vi "posctrl-drive-spin-sim.vi"(11 "Motor Demand":dbl) -> (3 "Rotation Change Deg":dbl)   [LabVIEW 2019]
uses:
  <vilib>/Rock Robotics/WPI/ThirdParty/JAS_Junk/TrajLib/LinearFilter_LP_BW1_Execute.vi
  <vilib>/Rock Robotics/WPI/ThirdParty/JAS_Junk/TrajLib/VI/TimeInterpDouble_New.vi
  <vilib>/Rock Robotics/WPI/ThirdParty/JAS_Junk/TrajLib/VI/TimeInterpDouble_AddSample.vi
  <vilib>/Rock Robotics/WPI/ThirdParty/JAS_Junk/TrajLib/VI/TimeInterpDouble_GetSample.vi
  <vilib>/Rock Robotics/WPI/ThirdParty/JAS_Junk/TrajLib/VI/TimeInterpDouble_SetMaxTime.vi
  <vilib>/Rock Robotics/WPI/ThirdParty/JAS_Junk/TrajLib/Util_GetTime.vi
  <vilib>/Rock Robotics/WPI/ThirdParty/JAS_Junk/TrajLib/LinearFilter_ResetToValue.vi
  <vilib>/Rock Robotics/WPI/ThirdParty/JAS_Junk/TrajLib/LinearFilter_Calculate.vi
  <vilib>/Rock Robotics/WPI/ThirdParty/JAS_Junk/TrajLib/VI/TimeInterpDouble_CleanUp.vi
  <vilib>/Rock Robotics/WPI/ThirdParty/JAS_Junk/TrajLib/MathUtil_Interpolate.vi
  <vilib>/Rock Robotics/WPI/ThirdParty/JAS_Junk/TrajLib/VI/Util_GetTime_U32.vi
  <vilib>/Rock Robotics/WPI/ThirdParty/JAS_Junk/TrajLib/VI/Util_GetTime_U64.vi
  <vilib>/gmath/interp.llb/Search Ordered Table.vi
  <vilib>/Rock Robotics/WPI/ThirdParty/JAS_Junk/TrajLib/LinearFilter_LowPassBW1.vi
  <vilib>/ptbypt/NI_PtbyPt.lvlib
  <vilib>/Rock Robotics/WPI/ThirdParty/JAS_Junk/TrajLib/Trajectory_Library.lvlib
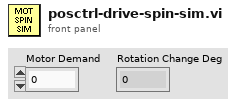
[diagram p1: front panel]
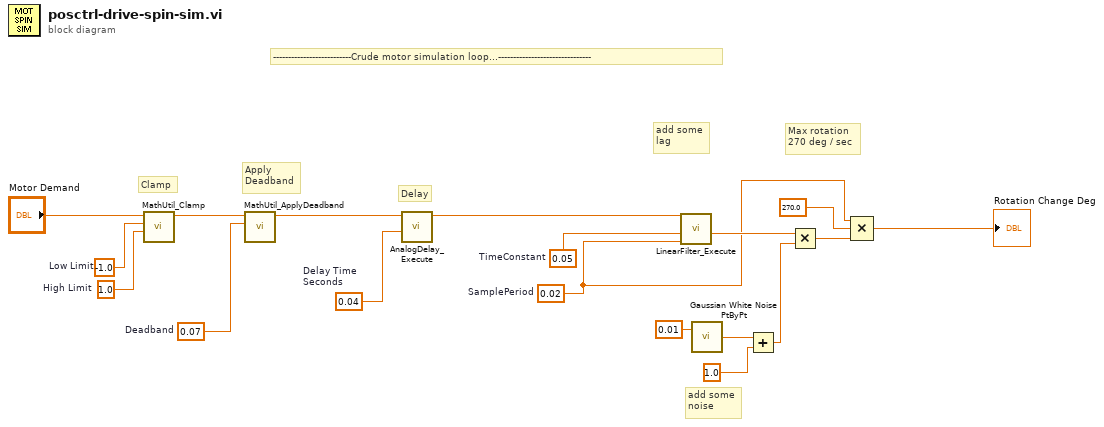
[diagram p0: block diagram]
diagram:
  w5 = 0.07  # Deadband
  w7 = 0.04  # Delay Time Seconds
  w10 = 1.0  # High Limit
  w9 = -1.0  # Low Limit
  w2 = 0.02  # SamplePeriod
  w1 = 0.05  # TimeConstant
  # "Apply\nDeadband"
  # "Delay"
  # "Max rotation \n270 deg / sec"
  # "Clamp"
  # "add some\nnoise"
  # "add some\nlag"
  # "--------------------------Crude motor simulation loop...-------------------------------"
  n1 = call <vilib>:"MathUtil_Clamp.vi"("High Limit"=w10, "Low Limit"=w9, "Value"="Motor Demand") -> ("Result"=w4:dbl)  [unwired: 8 in]
  n2 = call <vilib>:"MathUtil_ApplyDeadband.vi"("Deadband"=w5, "Value"=w4) -> ("Result"=w3:dbl)  [unwired: 9 in]
  n3 = call <vilib>:"AnalogDelay_Execute.vi"("Delay Time"=w7, "Input"=w3) -> ("Output"=w6:dbl)  [unwired: 8 in, 1 out]
  n4 = call-poly <vilib>:"LinearFilter_Execute.vi"("SamplePeriod"=w2, "TimeConstant"=w1, "Input"=w6) -> ("Output"=w14:dbl)  [unwired: 8 in]
  n5 = call <vilib>:"Gaussian White Noise PtByPt.vi"("standard deviation"=0.01) -> ("Gaussian white noise"=w15:dbl)  [unwired: 2 in]
  n6 = Add(x=w15, y=1.0) -> (x+y=w13:dbl)
  n7 = Multiply(x=w14, y=w13) -> (x*y=w12:dbl)
  n8 = Compound Arithmetic op=MULTIPLY(w2, 270.0 ("value"), w12) -> (→"Rotation Change Deg":dbl)
